vi "DEFINE_HMI.vi"() -> ()   [LabVIEW 2020]
uses:
  <vilib>/WebDAVClient/Advanced/Multi Event/Asynchronous Get File.vi
  Keyence CL-3000/Keyence CL-3000.lvlib
  <vilib>/WebDAVClient/NI_WebDAV.lvlib
panel:
  out "Index 1":u32
  out "Index 2":u32
  out "Data Points":u32
  in  "Log Chromatic Data":bool
  in  "stop":bool
  out "Camera Feed":T1(plugin-control)
  in  "Capture Image":bool
  out "Captured Image":T1(plugin-control)
  in  "Log Laser Data":bool
  out "Measurement Data":T2(array[cluster])=[{"Out No"=1, "Value"=0, "valueInfo"=enum."VALID", "judgeResult"=0}, {"Out No"=2, "Value"=0, "valueInfo"=enum."VALID", "judgeResult"=0}, {"Out No"=3, "Value"=0, "valueInfo"=enum."VALID", "judgeResult"=0}, {"Out No"=4, "Value"=0, "valueInfo"=enum."VALID", "judgeResult"=0}, {"Out No"=5, "Value"=0, "valueInfo"=enum."VALID", "judgeResult"=0}, {"Out No"=6, "Value"=0, "valueInfo"=enum."VALID", "judgeResult"=0}, {"Out No"=7, "Value"=0, "valueInfo"=enum."VALID", "judgeResult"=0}, {"Out No"=8, "Value"=0, "valueInfo"=enum."VALID", "judgeResult"=0}] {"judgeResult" items=["HI"=1, "GO"=2, "LO"=4, "**"=5, "--"=0]}
  in  "Save Location (Folder)":path
  in  "Test Name":string
  out "Laser Displacement Readings (cRIO)":dbl(graph)
  out "Chromatic Confocal Readings":dbl(graph)
  out "cRioTransferData":bool
  in  "Comm Interface":enum8{"USB", "ETHERNET"}(ring)
  in  "Device ID":i32 min=0 max=2
  in  "IP Address":u8[](array[numeric])=[192, 168, 1, 1]
  in  "Port":u32
  in  "timeout":u32=5000 caption="Timeout"
  out "Chromatic Confocal":errorcluster {"code" format="%x"}
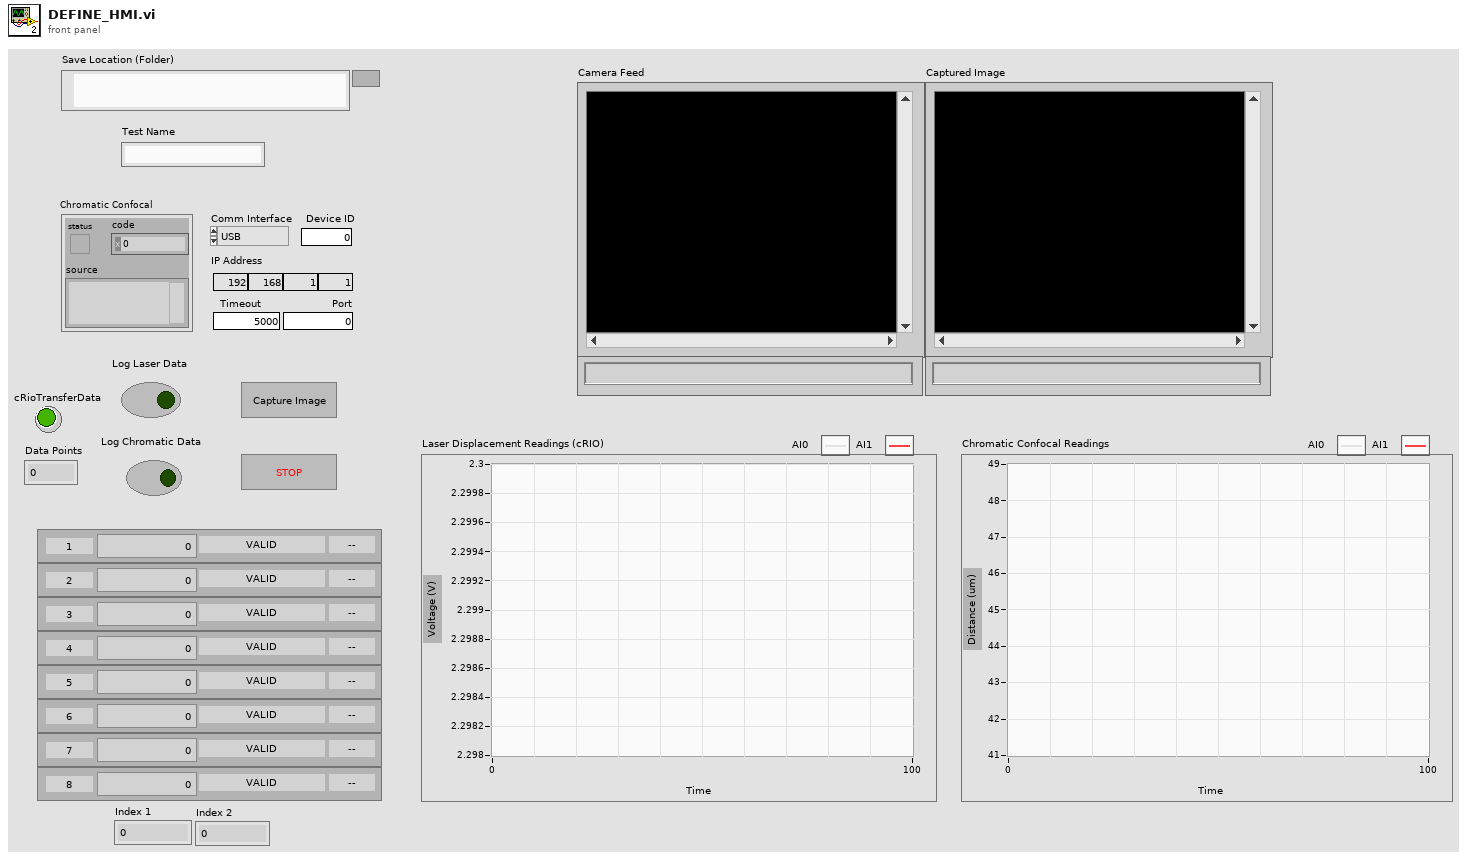
[diagram p1: front panel]
types:
  T1 = typedef "IMAQ Image.ctl" = refnum<image>
  T2 = cluster{"Out No":i32, "Value":i32, "valueInfo":enum8{"VALID", "JUDGMENTSTANDBY", "INVALID", "OVERDISPRANGE_P", "OVERDISPRANGE_N"}, "judgeResult":u16}[]
  T3 = enum16{"open", "replace", "create", "open or create", "replace or create", "replace or create with confirmation"}
  T4 = typedef "Keyence CL-3000.lvlib/CL3IF_MEASUREMENT_DATA.ctl" = cluster{"addInfo":cluster{"triggerCount":u32, "pulseCount":i32}, "outMeasurementData":T5[]}
  T5 = typedef "Keyence CL-3000.lvlib/CL3IF_OUTMEASUREMENT_DATA.ctl" = cluster{"measurementValue":i32, "valueInfo":T6, "judgeResult":T7}
  T6 = typedef "Keyence CL-3000.lvlib/CL3IF_VALUE_INFO.ctl" = enum8{"VALID", "JUDGMENTSTANDBY", "INVALID", "OVERDISPRANGE_P", "OVERDISPRANGE_N"}
  T7 = typedef "Keyence CL-3000.lvlib/CL3IF_JUDGE_RESULT.ctl" = u8
  T8 = cluster{i32, "measurementValue":i32, "valueInfo":T6, "judgeResult":T7}
  T9 = typedef "NI_WebDAV.lvlib/Asynchronous Session Handle.ctl" = refnum<k1>
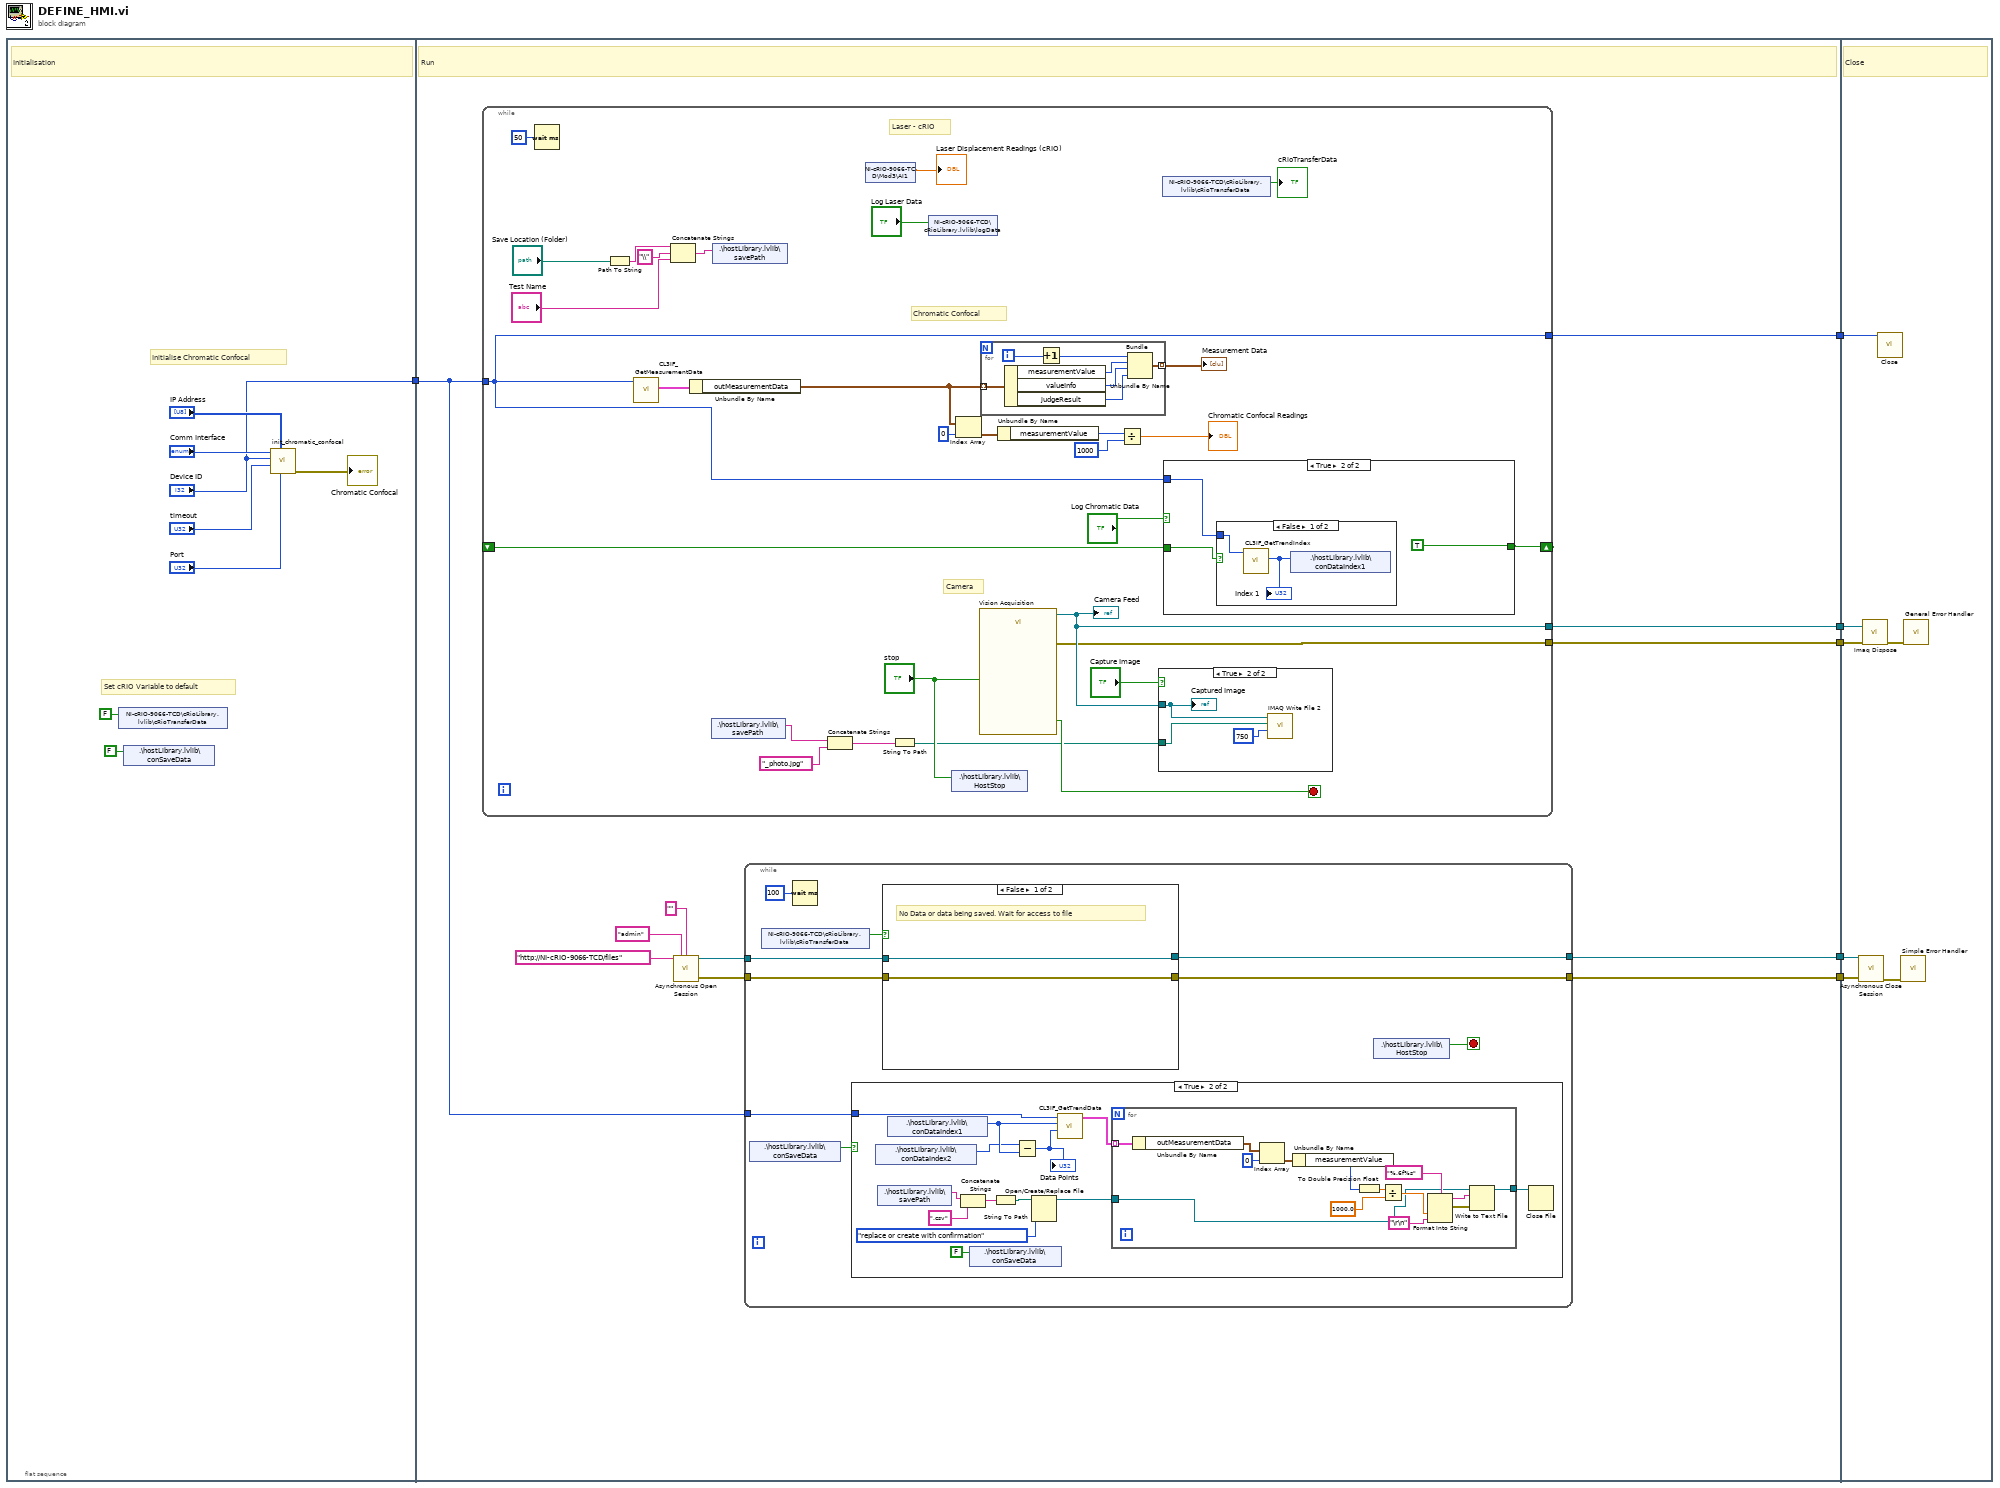
[diagram p0: block diagram]
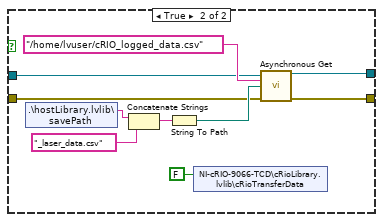
[diagram p3: hidden frame]
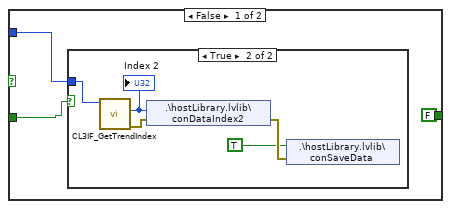
[diagram p4: hidden frame]
diagram:
  n1 = flat-sequence {
    tunnel: ["Device ID"] -> w6
    tunnel: w6 -> [w15]
    tunnel: [w25] -> w5
    tunnel: [w24] -> w4
    tunnel: [w23] -> w3
    tunnel: [w17] -> w2
    tunnel: [w16] -> w1
    tunnel: w5 -> [w132]
    tunnel: w4 -> [w131]
    tunnel: w3 -> [w130]
    tunnel: w2 -> [w128]
    tunnel: w1 -> [w127]
    frame #0 {
      # "Set cRIO Variable to default"
      # "Initialise Chromatic Confocal"
      # "Initialisation"
      n2 = shared-variable "NI-cRIO-9066-TCD\\cRioLibrary.lvlib\\cRioTransferData"(FALSE ("cRioTransferData")) -> ()  [unwired: 1 in, 1 out]
      n3 = shared-variable ".\\hostLibrary.lvlib\\conSaveData"(FALSE ("conSaveData")) -> ()  [unwired: 1 in, 1 out]
      n4 = call "init_chromatic_confocal.vi"("Port"="Port", "IP Address"="IP Address", "timeout"="timeout", "Device ID"="Device ID", "Comm Interface"="Comm Interface") -> ("error out"=→"Chromatic Confocal":errorcluster)  [unwired: 6 in]
    }
    frame #1 {
      # "Run"
      n5 = while {
        tunnel: [w100] -> w25
        tunnel: [w99] -> w24
        tunnel: w15 -> [w85]
        tunnel: [w85] -> w23
        shift-right: [w83] -> _
        shift-left: _ -> [w82]
        stop <- w102 stop-if-true
        # "Camera"
        # "Chromatic Confocal"
        # "Laser - cRIO"
        n6 = Wait (ms)(milliseconds to wait=u32 50) -> ()  [unwired: 1 out]
        n7 = Path To String(path="Save Location (Folder)") -> (string=w80:string)
        n8 = call "CL3IF_GetMeasurementData.vi"("deviceId"=w85) -> ("MEASUREMENT_DATA"=w97:T4)  [unwired: 9 in, 1 out]
        n9 = Concatenate Strings(w80, "\\" ("string"), "Test Name") -> (w79:string)
        n10 = Unbundle By Name(w97) -> ("outMeasurementData"=w95:T5[])
        n11 = shared-variable ".\\hostLibrary.lvlib\\savePath"() -> (w78:string)  [unwired: 1 in, 1 out]
        n12 = shared-variable ".\\hostLibrary.lvlib\\savePath"(w79) -> ()  [unwired: 1 in, 1 out]
        n13 = Concatenate Strings(w78, "_photo.jpg" ("string")) -> (w77:string)
        n14 = shared-variable "NI-cRIO-9066-TCD\\Mod3\\AI1"() -> (→"Laser Displacement Readings (cRIO)":dbl)  [unwired: 1 in, 1 out]
        n15 = String To Path(string=w77) -> (path=w76:path)
        n16 = shared-variable "NI-cRIO-9066-TCD\\cRioLibrary.lvlib\\logData"("Log Laser Data") -> ()  [unwired: 1 in, 1 out]
        n17 = shared-variable ".\\hostLibrary.lvlib\\HostStop"("stop") -> ()  [unwired: 1 in, 1 out]
        n18 = Index Array(array=w95, index=0) -> (element=w94:T5)
        n19 = call "Vision Acquisition"("Stop (F)"="stop") -> ("Image Out"=w100:T1, "Stopped"=w102:bool, "error out"=w99:errorcluster)  [unwired: 1 in, 23 out]
        "Camera Feed" <- w100
        n20 = for {
          tunnel: w95 -> [w123] mode=indexing
          tunnel: [w122] -> w98 mode=indexing
          i -> [w121]
          n21 = Unbundle By Name(w123) -> ("measurementValue"=w117:i32, "valueInfo"=w119:T6, "judgeResult"=w118:T7)
          n22 = Increment(x=w121) -> (x+1=w120:i32)
          n23 = Bundle(w120, "measurementValue"=w117, "valueInfo"=w119, "judgeResult"=w118) -> (w122:T8)  [unwired: 1 in]
        }
        "Measurement Data" <- w98
        n24 = Unbundle By Name(w94) -> ("measurementValue"=w93:i32)
        n25 = Divide(x=w93, y=1000) -> (x/y=→"Chromatic Confocal Readings":dbl)
        n26 = case shown="True" "Capture Image" {
          tunnel: w100 -> [_ w126]
          tunnel: w76 -> [_ w124]
          frame False {
          }
          frame True {
            n27 = call-poly "IMAQ Write File 2"("Image Quality"=u32 750, "File Path"=w124, "Image"=w126) -> ()  [unwired: 7 in, 2 out]
            "Captured Image" <- w126
          }
        }
        n28 = shared-variable "NI-cRIO-9066-TCD\\cRioLibrary.lvlib\\cRioTransferData"() -> (→"cRioTransferData":bool)  [unwired: 1 in, 1 out]
        n29 = case shown="True" "Log Chromatic Data" {
          tunnel: w85 -> [w104 w112]
          tunnel: [FALSE TRUE] -> w83
          tunnel: w82 -> [w105 w113]
          frame False {
            n30 = case shown="True" w105 {
              tunnel: w104 -> [_ w111]
              frame False {
                # "do nothing"
              }
              frame True {
                n31 = call "CL3IF_GetTrendIndex.vi"("deviceId"=w111) -> ("error out"=w107:errorcluster, "index"=w110:u32)  [unwired: 9 in]
                "Index 2" <- w110
                n32 = shared-variable ".\\hostLibrary.lvlib\\conDataIndex2"(w110, error in=w107) -> (error out=w109:errorcluster)
                n33 = shared-variable ".\\hostLibrary.lvlib\\conSaveData"(TRUE ("conSaveData"), error in=w109) -> ()  [unwired: 1 out]
              }
            }
          }
          frame True {
            n34 = case shown="False" w113 {
              tunnel: w112 -> [w116 _]
              frame False {
                n35 = call "CL3IF_GetTrendIndex.vi"("deviceId"=w116) -> ("index"=w115:u32)  [unwired: 9 in, 1 out]
                "Index 1" <- w115
                n36 = shared-variable ".\\hostLibrary.lvlib\\conDataIndex1"(w115) -> ()  [unwired: 1 in, 1 out]
              }
              frame True {
                # "Do nothing"
              }
            }
          }
        }
      }
      n37 = call <vilib>:"Asynchronous Open Session.vi"("host uri prefix"="http://NI-cRIO-9066-TCD/files", "username"="admin", "password"="") -> ("session handle out"=w19:T9, "error out"=w18:errorcluster)  [unwired: 10 in, 1 out]
      n38 = while {
        tunnel: w19 -> [w32]
        tunnel: w18 -> [w31]
        tunnel: [w30] -> w17
        tunnel: [w29] -> w16
        tunnel: w15 -> [w26]
        stop <- w28 stop-if-true
        n39 = shared-variable ".\\hostLibrary.lvlib\\conSaveData"() -> (w27:bool)  [unwired: 1 in, 1 out]
        n40 = shared-variable "NI-cRIO-9066-TCD\\cRioLibrary.lvlib\\cRioTransferData"() -> (w34:bool)  [unwired: 1 in, 1 out]
        n41 = Wait (ms)(milliseconds to wait=u32 100) -> ()  [unwired: 1 out]
        n42 = case shown="True" w27 {
          tunnel: w26 -> [_ w45]
          frame False {
            # "Do Nothing"
          }
          frame True {
            n43 = shared-variable ".\\hostLibrary.lvlib\\conDataIndex2"() -> (w35:u32)  [unwired: 1 in, 1 out]
            n44 = shared-variable ".\\hostLibrary.lvlib\\savePath"() -> (w38:string)  [unwired: 1 in, 1 out]
            n45 = shared-variable ".\\hostLibrary.lvlib\\conDataIndex1"() -> (w36:u32)  [unwired: 1 in, 1 out]
            n46 = Concatenate Strings(w38, ".csv" ("string")) -> (w42:string)
            n47 = shared-variable ".\\hostLibrary.lvlib\\conSaveData"(FALSE ("conSaveData")) -> ()  [unwired: 1 in, 1 out]
            n48 = String To Path(string=w42) -> (path=w41:path)
            n49 = Subtract(x=w35, y=w36) -> (x-y=w46:u32)
            "Data Points" <- w46
            n50 = Open/Create/Replace File(file path (use dialog)=w41, operation (0:open)=T3."replace or create with confirmation") -> (refnum out=w40:refnum<file>)  [unwired: 4 in, 2 out]
            n51 = call "CL3IF_GetTrendData.vi"("requestDataCount"=w46, "index"=w36, "deviceId"=w45) -> ("measurementData"=w44:T4[])  [unwired: 4 in, 4 out]
            n52 = for {
              tunnel: w44 -> [w61] mode=indexing
              tunnel: w40 -> [w50]
              tunnel: [w48] -> w39
              n53 = Unbundle By Name(w61) -> ("outMeasurementData"=w59:T5[])
              n54 = Index Array(array=w59, index=0) -> (element=w58:T5)
              n55 = Unbundle By Name(w58) -> ("measurementValue"=w55:i32)
              n56 = To Double Precision Float(number=w55) -> (double precision float=w56:dbl)
              n57 = Divide(x=w56, y=1000.0) -> (x/y=w54:dbl)
              n58 = Format Into String(format string="%.6f%s", w54, "\r\n") -> (resulting string=w51:string, error out=w49:errorcluster)  [unwired: 2 in]
              n59 = Write to Text File(file (use dialog)=w50, text=w51, error in=w49) -> (refnum out=w48:refnum<file>)  [unwired: 1 in, 2 out]
            }
            n60 = Close File(refnum=w39) -> ()  [unwired: 1 in, 2 out]
          }
        }
        n61 = case shown="False" w34 {
          tunnel: w32 -> [w63 w71]
          tunnel: w31 -> [w62 w70]
          tunnel: [w63 w69] -> w30
          tunnel: [w62 w68] -> w29
          frame False {
            # "No Data or data being saved. Wait for access to file"
          }
          frame True {
            n62 = shared-variable ".\\hostLibrary.lvlib\\savePath"() -> (w65:string)  [unwired: 1 in, 1 out]
            n63 = Concatenate Strings(w65, "_laser_data.csv" ("string")) -> (w67:string)
            n64 = String To Path(string=w67) -> (path=w73:path)
            n65 = shared-variable "NI-cRIO-9066-TCD\\cRioLibrary.lvlib\\cRioTransferData"(FALSE ("cRioTransferData")) -> ()  [unwired: 1 in, 1 out]
            n66 = call-poly <vilib>:"Asynchronous Get.vi"("session handle"=w71, "relative uri"="/home/lvuser/cRIO_logged_data.csv", "local file path"=w73, "error in (no error)"=w70) -> ("session handle out"=w69:T9, "error out"=w68:errorcluster)  [unwired: 8 in, 2 out]
          }
        }
        n67 = shared-variable ".\\hostLibrary.lvlib\\HostStop"() -> (w28:bool)  [unwired: 1 in, 1 out]
      }
    }
    frame #2 {
      # "Close"
      n68 = call <vilib>:"Asynchronous Close Session.vi"("session handle"=w128, "error in (no error)"=w127) -> ("error out"=w129:errorcluster)  [unwired: 13 in]
      n69 = call "Imaq Dispose"("Image"=w132, "error in (no error)"=w131) -> ("error out"=w133:errorcluster)  [unwired: 4 in]
      n70 = call "Close.vi"("deviceId"=w130) -> ()  [unwired: 10 in, 1 out]
      n71 = call <vilib>:"Simple Error Handler.vi"("error in (no error)"=w129) -> ()  [unwired: 4 in, 5 out]
      n72 = call <vilib>:"General Error Handler.vi"("error in (no error)"=w133) -> ()  [unwired: 2 in, 13 out]
    }
  }
